vi "Proiect VREME.vi"() -> ()   [LabVIEW 2020]
panel:
  out "SENIN":bool
  out "SECETA":bool
  out "NINSOARE":bool
  out "PLOAIE":bool
  in  "Indicator PRAF":dbl(slide) scale=0.0..10.0
  in  "Indicator TEMPERATURA":dbl(slide) scale=-20.0..50.0
  in  "Indicator UMIDITATE":dbl(slide) scale=0.0..100.0
  out "Umiditate(%)":dbl(knob) scale=0.0..100.0
  out "Materie (grame)":dbl
  out "Temperatura (°C)":dbl(slide) scale=-20.0..50.0
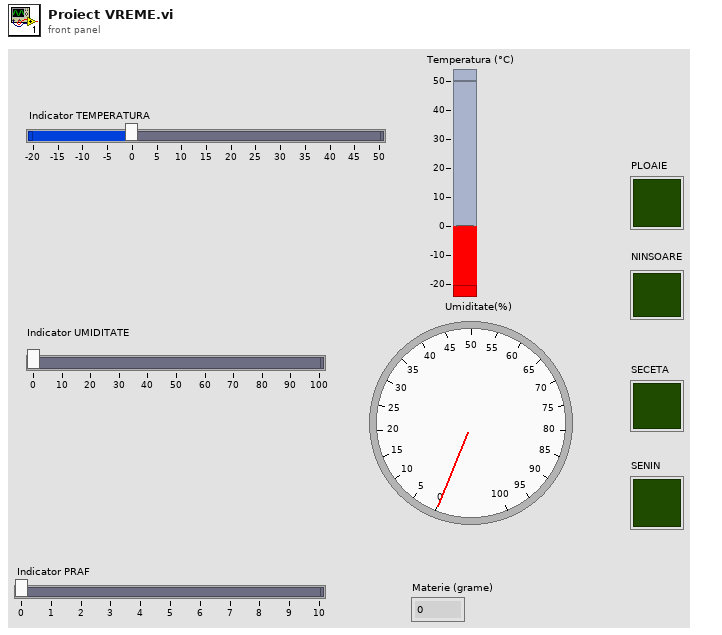
[diagram p1: front panel]
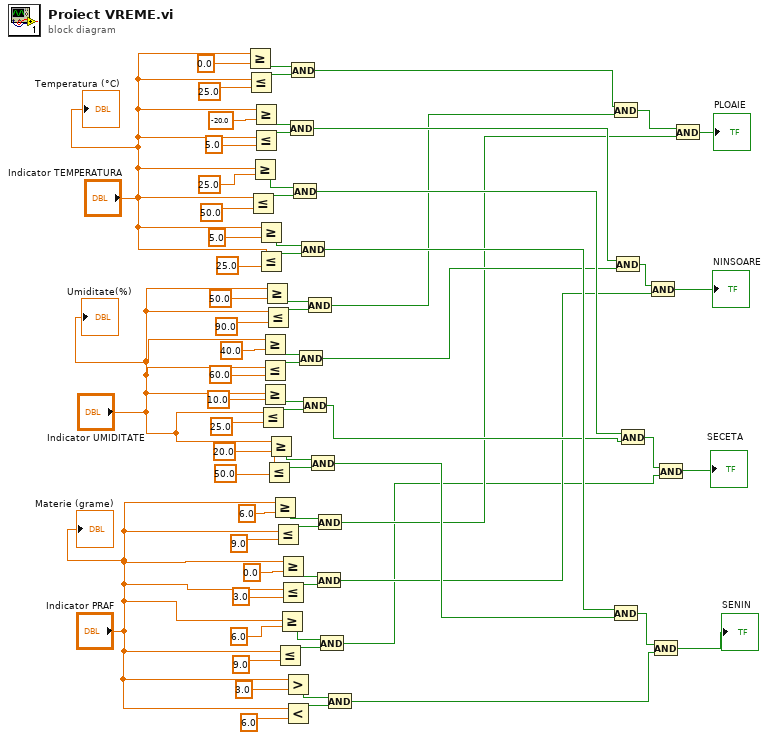
[diagram p0: block diagram]
diagram:
  n1 = Greater Or Equal?(x="Indicator TEMPERATURA", y=0.0) -> (x >= y?=w71:bool)
  n2 = Less Or Equal?(x="Indicator TEMPERATURA", y=25.0) -> (x <= y?=w70:bool)
  n3 = Less Or Equal?(x="Indicator TEMPERATURA", y=50.0) -> (x <= y?=w62:bool)
  n4 = Greater Or Equal?(x="Indicator TEMPERATURA", y=25.0) -> (x >= y?=w63:bool)
  n5 = Greater Or Equal?(x="Indicator TEMPERATURA", y=-20.0) -> (x >= y?=w64:bool)
  n6 = Less Or Equal?(x="Indicator TEMPERATURA", y=5.0) -> (x <= y?=w65:bool)
  n7 = Greater Or Equal?(x="Indicator TEMPERATURA", y=5.0) -> (x >= y?=w56:bool)
  n8 = Less Or Equal?(x="Indicator TEMPERATURA", y=25.0) -> (x <= y?=w57:bool)
  n9 = Less Or Equal?(x="Indicator UMIDITATE", y=25.0) -> (x <= y?=w48:bool)
  n10 = Greater Or Equal?(x="Indicator UMIDITATE", y=40.0) -> (x >= y?=w46:bool)
  n11 = Less Or Equal?(x="Indicator UMIDITATE", y=60.0) -> (x <= y?=w45:bool)
  n12 = Greater Or Equal?(x="Indicator UMIDITATE", y=10.0) -> (x >= y?=w47:bool)
  n13 = Greater Or Equal?(x="Indicator UMIDITATE", y=50.0) -> (x >= y?=w39:bool)
  n14 = Less Or Equal?(x="Indicator UMIDITATE", y=90.0) -> (x <= y?=w40:bool)
  n15 = Less Or Equal?(x="Indicator UMIDITATE", y=50.0) -> (x <= y?=w53:bool)
  n16 = Greater Or Equal?(x="Indicator UMIDITATE", y=20.0) -> (x >= y?=w54:bool)
  n17 = Greater Or Equal?(x="Indicator PRAF", y=6.0) -> (x >= y?=w38:bool)
  n18 = Less Or Equal?(x="Indicator PRAF", y=9.0) -> (x <= y?=w37:bool)
  n19 = Less Or Equal?(x="Indicator PRAF", y=9.0) -> (x <= y?=w29:bool)
  n20 = Greater Or Equal?(x="Indicator PRAF", y=6.0) -> (x >= y?=w30:bool)
  n21 = Greater Or Equal?(x="Indicator PRAF", y=0.0) -> (x >= y?=w31:bool)
  n22 = Less Or Equal?(x="Indicator PRAF", y=3.0) -> (x <= y?=w32:bool)
  n23 = Greater?(x="Indicator PRAF", y=3.0) -> (0:w23:bool)
  n24 = Less?(x="Indicator PRAF", y=6.0) -> (x < y?=w24:bool)
  n25 = And(x=w64, y=w65) -> (x .and. y?=w11:bool)
  n26 = And(x=w71, y=w70) -> (x .and. y?=w12:bool)
  n27 = And(x=w63, y=w62) -> (x .and. y?=w10:bool)
  n28 = And(x=w46, y=w45) -> (x .and. y?=w7:bool)
  n29 = And(x=w56, y=w57) -> (x .and. y?=w9:bool)
  n30 = And(x=w47, y=w48) -> (x .and. y?=w6:bool)
  n31 = And(x=w39, y=w40) -> (x .and. y?=w8:bool)
  n32 = And(x=w54, y=w53) -> (x .and. y?=w5:bool)
  n33 = And(x=w31, y=w32) -> (x .and. y?=w3:bool)
  n34 = And(x=w38, y=w37) -> (x .and. y?=w4:bool)
  n35 = And(x=w30, y=w29) -> (x .and. y?=w2:bool)
  n36 = And(x=w23, y=w24) -> (x .and. y?=w1:bool)
  n37 = And(x=w12, y=w8) -> (x .and. y?=w20:bool)
  n38 = And(x=w9, y=w5) -> (x .and. y?=w18:bool)
  n39 = And(x=w11, y=w7) -> (x .and. y?=w19:bool)
  n40 = And(x=w10, y=w6) -> (x .and. y?=w17:bool)
  n41 = And(x=w19, y=w3) -> (x .and. y?=→"NINSOARE":bool)
  n42 = And(x=w18, y=w1) -> (x .and. y?=→"SENIN":bool)
  n43 = And(x=w17, y=w2) -> (x .and. y?=→"SECETA":bool)
  n44 = And(x=w20, y=w4) -> (x .and. y?=→"PLOAIE":bool)
  "Temperatura (°C)" <- "Indicator TEMPERATURA"
  "Materie (grame)" <- "Indicator PRAF"
  "Umiditate(%)" <- "Indicator UMIDITATE"
